vi "FPGA_measure_QPD_signal.vi"() -> ()   [LabVIEW 2015]
uses:
  <vilib>/Platform/TimedLoop/XDataNode/timing_clust.ctl
  <vilib>/Platform/TimedLoop/XDataNode/nitl_modes.ctl
  <vilib>/Platform/TimedLoop/XDataNode/wakeup.ctl
  <vilib>/rvi/FXPMathLib/basic elements/FxpIntAccumulator/subVIs/nifxpmath_IntAccumulator_SimConfig.ctl
  <vilib>/rvi/Emulation/niFpgaGetClockAttributes.vi
  <vilib>/rvi/Emulation/niFpgaSctlEmulationGetInTimedLoop.vi
  <vilib>/rvi/Emulation/niFpgaEmulationReportErrorSimple.vi
  <vilib>/rvi/Emulation/niFpgaProcessEmulError.vi
  <vilib>/rvi/eio/common/nirviEmuTemplateMethod_errors.vi
  <vilib>/rvi/Analysis/common/codeGenErrors/XNode/niFpgaXNodeCodeGenErrorHandle.vi
  <vilib>/rvi/Emulation/niFpgaCriticalErrorInLSC.vi
  <vilib>/rvi/FXPMathLib/basic elements/FxpIntAccumulator/simVIs/DllFxpIntAccumulator_sub.vi
  <vilib>/eio/EIONode/EIONode.xnode
  <vilib>/rvi/Analysis/measure/dc-rms/XNode/niFpgaDC-RMS.xnode
  <vilib>/Platform/TimedLoop/XDataNode/XDataNode.xnode
  <vilib>/rvi/FXPMathLib/basic elements/FxpIntAccumulator/XNode/nifxpmath_IntAccumulator.xnode
  <vilib>/Platform/TimedLoop/XDataNode/XDNodeRunTimeDep.lvlib
panel:
  in  "561":sgl
  in  "640":sgl
  in  "405":sgl
  in  "488":sgl
  in  "Update lasers":bool
  in  "Reset counter":bool
  out "QPD":T1
  in  "Count(uSec)":u32=100
  out "duration (ms)":u32
  in  "stop":bool
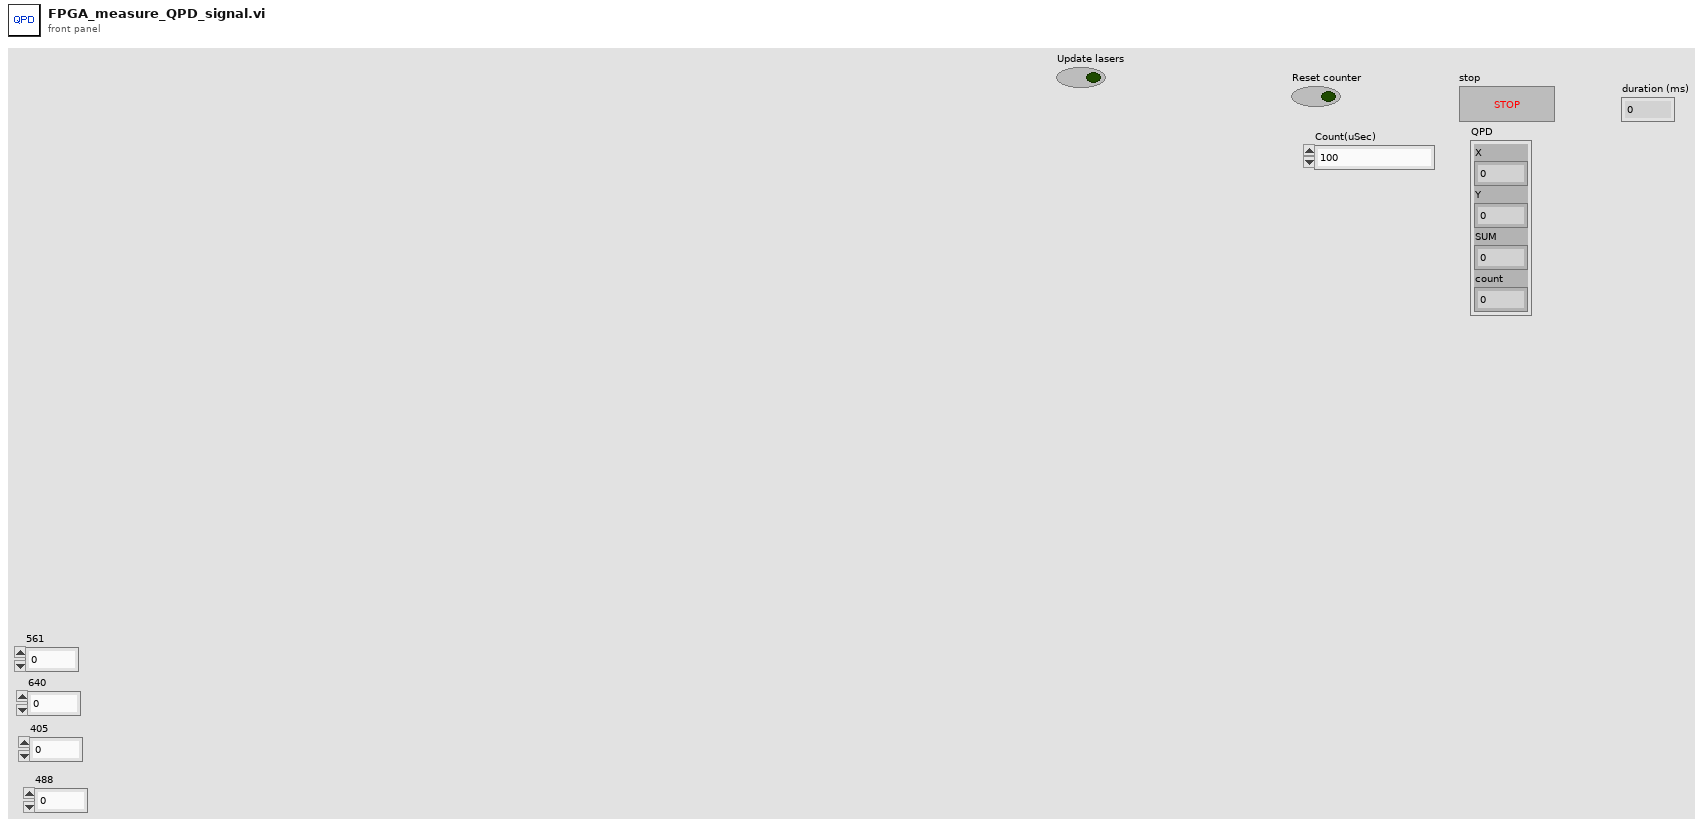
[diagram p1: front panel]
types:
  T1 = cluster{"X":sgl, "Y":sgl, "SUM":sgl, "count":u32}
  T2 = typedef "XDNodeRunTimeDep.lvlib/timing_clust.ctl" = cluster{"Expected End [f-1]":u64, "Actual End [f-1]":u64, "Finished Late? [f-1]":bool, "Expected End [i-1]":u64, "Actual End [i-1]":u64, "Finished Late? [i-1]":bool, "Expected Start [i]":u64, "Actual Start [i]":u64, "Expected Start [f]":u64, "Actual Start [f]":u64, "Source Name":string, "Structure Name":string, "Period":i64, "Deadline":i64, "Offset":i64, "Start":i64, "Priority":i32, "Timeout":i32, "Mode":T3, "Wakeup Reason":T4, "Error":errorcluster, "Source Type":string, "Secondary Source Type":string, "Global End Time":u64, "Global Start Time":u64, "Frame Duration":u64, "Iteration Duration":u64, "Assigned CPU":i32, "I/O Scan Engine Mode":u32}
  T3 = typedef "XDNodeRunTimeDep.lvlib/nitl_modes.ctl" = enum32{"No Change", "Process missed periods, maintain original phase", "Discard missed periods, maintain original phase", "Process missed periods, ignore original phase", "Discard missed periods, ignore original phase"}
  T4 = typedef "XDNodeRunTimeDep.lvlib/wakeup.ctl" = enum32{"Normal", "Aborted", "Asynchronous wakeup", "Timing source error", "Timed loop error", "Timeout"}
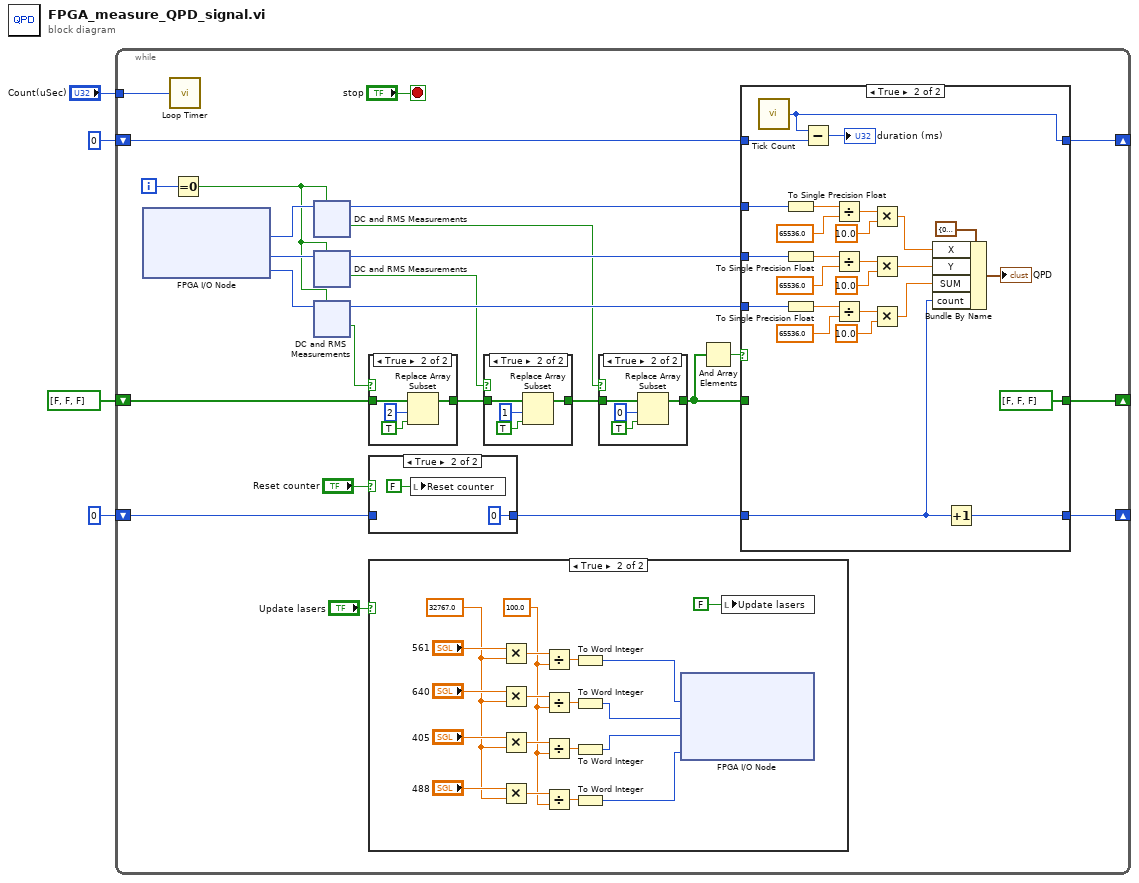
[diagram p0: block diagram]
diagram:
  n1 = while {
    shift-right: [w13] -> _
    shift-left: bool[] [FALSE, FALSE, FALSE] ("initialized array") -> [w21]
    shift-right: [w11] -> _
    shift-left: u32 0 -> [w12]
    tunnel: "Count(uSec)" -> [w10]
    shift-right: [w9] -> _
    shift-left: u32 0 -> [w7]
    i -> [w28]
    stop <- "stop" stop-if-true
    n2 = xnode "FPGA I/O Node"() -> ("Connector0/AI0"=w30:i16, "Connector0/AI1"=w26:i16, "Connector0/AI2"=w25:i16)  [unwired: 3 in, 3 out]
    n3 = call "Loop Timer"("Count(uSec)"=w10) -> ()  [unwired: 1 out]
    n4 = Equal To 0?(x=w28) -> (x = 0?=w22:bool)
    n5 = xnode "DC and RMS Measurements"("input data"=w30, "reset"=w22) -> ("DC"=w27:i16, "output valid"=w16:bool)
    n6 = xnode "DC and RMS Measurements"("input data"=w26, "reset"=w22) -> ("DC"=w24:i16, "output valid"=w17:bool)
    n7 = xnode "DC and RMS Measurements"("input data"=w25, "reset"=w22) -> ("DC"=w23:i16, "output valid"=w18:bool)
    n8 = case shown="True" w18 {
      tunnel: w21 -> [w58 w61]
      tunnel: [w58 w59] -> w20
      frame False {
      }
      frame True {
        n9 = Replace Array Subset(array=w61, new element=TRUE, index=2) -> (w59:bool[])
      }
    }
    n10 = case shown="True" "Reset counter" {
      tunnel: w7 -> [w50 _]
      tunnel: [w50 u32 0] -> w6
      frame False {
      }
      frame True {
        n11 = local write "Reset counter"(FALSE ("Reset counter")) -> ()
      }
    }
    n12 = case shown="True" "Update lasers" {
      frame False {
      }
      frame True {
        w33 = sgl 100.0
        w34 = sgl 32767.0
        n13 = Multiply(x="561", y=w34) -> (x*y=w48:sgl)
        n14 = Multiply(x="640", y=w34) -> (x*y=w44:sgl)
        n15 = Multiply(x="405", y=w34) -> (x*y=w40:sgl)
        n16 = Multiply(x="488", y=w34) -> (x*y=w36:sgl)
        n17 = Divide(x=w48, y=w33) -> (x/y=w47:sgl)
        n18 = Divide(x=w44, y=w33) -> (x/y=w45:sgl)
        n19 = Divide(x=w40, y=w33) -> (x/y=w39:sgl)
        n20 = Divide(x=w36, y=w33) -> (x/y=w37:sgl)
        n21 = To Word Integer(number=w47) -> (16bit integer=w46:i16)
        n22 = To Word Integer(number=w45) -> (16bit integer=w42:i16)
        n23 = To Word Integer(number=w39) -> (16bit integer=w38:i16)
        n24 = To Word Integer(number=w37) -> (16bit integer=w32:i16)
        n25 = xnode "FPGA I/O Node"("Connector0/AO0"=w46, "Connector0/AO1"=w42, "Connector0/AO2"=w38, "Connector0/AO3"=w32) -> ()  [unwired: 4 in, 4 out]
        n26 = local write "Update lasers"(FALSE ("Update lasers")) -> ()
      }
    }
    n27 = case shown="True" w17 {
      tunnel: w20 -> [w63 w66]
      tunnel: [w63 w64] -> w19
      frame False {
      }
      frame True {
        n28 = Replace Array Subset(array=w66, new element=TRUE, index=1) -> (w64:bool[])
      }
    }
    n29 = case shown="True" w16 {
      tunnel: [w53 w55] -> w14
      tunnel: w19 -> [w53 w54]
      frame False {
      }
      frame True {
        n30 = Replace Array Subset(array=w54, new element=TRUE, index=0) -> (w55:bool[])
      }
    }
    n31 = And Array Elements(Boolean array=w14) -> (logical AND=w15:bool)
    n32 = case shown="True" w15 {
      tunnel: w27 -> [_ w96]
      tunnel: w24 -> [_ w87]
      tunnel: w23 -> [_ w82]
      tunnel: w14 -> [w70 _]
      tunnel: [w70 bool[] [FALSE, FALSE, FALSE] ("initialized array")] -> w13
      tunnel: w12 -> [w69 w77]
      tunnel: [w69 w75] -> w11
      tunnel: w6 -> [w68 w72]
      tunnel: [w68 w71] -> w9
      frame False {
      }
      frame True {
        n33 = call "Tick Count"() -> ("Tick Count(mSec)"=w75:u32)
        n34 = To Single Precision Float(number=w96) -> (single precision float=w95:sgl)
        n35 = To Single Precision Float(number=w87) -> (single precision float=w88:sgl)
        n36 = To Single Precision Float(number=w82) -> (single precision float=w86:sgl)
        n37 = Subtract(x=w75, y=w77) -> (x-y=→"duration (ms)":u32)
        n38 = Divide(x=w95, y=sgl 65536.0) -> (x/y=w93:sgl)
        n39 = Divide(x=w88, y=sgl 65536.0) -> (x/y=w90:sgl)
        n40 = Divide(x=w86, y=sgl 65536.0) -> (x/y=w84:sgl)
        n41 = Multiply(x=w93, y=sgl 10.0) -> (x*y=w81:sgl)
        n42 = Multiply(x=w90, y=sgl 10.0) -> (x*y=w80:sgl)
        n43 = Multiply(x=w84, y=sgl 10.0) -> (x*y=w79:sgl)
        n44 = Bundle By Name(cluster=T1 {"X"=0.0, "Y"=0.0, "SUM"=0.0, "count"=0} ("output cluster"), "X"=w81, "Y"=w80, "SUM"=w79, "count"=w72) -> (→"QPD":T1)
        n45 = Increment(x=w72) -> (x+1=w71:u32)
      }
    }
  }
